vi "Sample 3 - Async Programming.vi"() -> ()   [LabVIEW 2016]
panel:
  in  "System Locator":string="usb:ix:0"
  in  "exit":bool
  out "Error":errorcluster
  out "Status B":T1(ring)
  out "Status A":T1(ring)
  in  "Channel B":u32
  in  "Channel A":u32
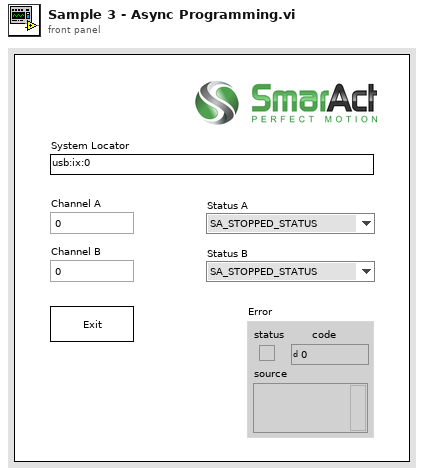
[diagram p1: front panel]
types:
  T1 = enum16{"SA_STOPPED_STATUS", "SA_STEPPING_STATUS", "SA_SCANNING_STATUS", "SA_HOLDING_STATUS", "SA_TARGET_STATUS", "SA_MOVE_DELAY_STATUS", "SA_CALIBRATING_STATUS", "SA_FINDING_REF_STATUS", "SA_OPENING_STATUS"}
  T2 = enum32{"SA_UNBUFFERED_OUTPUT", "SA_BUFFERED_OUTPUT"}
  T3 = typedef "mcsPacket.ctl" = cluster{"packetType":enum32{"SA_NO PACKET_TYPE", "SA_ERROR_ PACKET_TYPE", "SA_POSITION PACKET_TYPE", "SA_COMPLETED PACKET_TYPE", "SA_STATUS PACKET_TYPE", "SA_ANGLE_PACKET_TYPE", "SA_VOLTAGE_LEVEL_PACKET_TYPE", "SA_SENSOR_TYPE_PACKET_TYPE", "SA_SENSOR_ENABLED_PACKET_TYPE", "SA_END_EFFECTOR_TYPE_PACKET_TYPE", "SA_GRIPPER_OPENING_PACKET_TYPE", "SA_FORCE_PACKET_TYPE", "SA_MOVE_SPEED_PACKET_TYPE", "SA_PHYSICAL_POSITION_KNOWN_PACKET_TYPE", "SA_POSITION_LIMIT_PACKET_TYPE", "SA_ANGLE_LIMIT_PACKET_TYPE", "SA_SAFE_DIRECTION_PACKET_TYPE", "SA_SCALE_PACKET_TYPE", "SA_MOVE_ACCELERATION_PACKET_TYPE", "SA_CHANNEL_PROPERTY_PACKET_TYPE", "SA_CAPTURE_BUFFER_PACKET_TYPE", "SA_TRIGGERED_PACKET_TYPE"}, "channelIndex":u32, "data1":u32, "data2":i32, "data3":i32, "data4":u32}
  T4 = enum32{"SA_NO PACKET_TYPE", "SA_ERROR_ PACKET_TYPE", "SA_POSITION PACKET_TYPE", "SA_COMPLETED PACKET_TYPE", "SA_STATUS PACKET_TYPE", "SA_ANGLE_PACKET_TYPE", "SA_VOLTAGE_LEVEL_PACKET_TYPE", "SA_SENSOR_TYPE_PACKET_TYPE", "SA_SENSOR_ENABLED_PACKET_TYPE", "SA_END_EFFECTOR_TYPE_PACKET_TYPE", "SA_GRIPPER_OPENING_PACKET_TYPE", "SA_FORCE_PACKET_TYPE", "SA_MOVE_SPEED_PACKET_TYPE", "SA_PHYSICAL_POSITION_KNOWN_PACKET_TYPE", "SA_POSITION_LIMIT_PACKET_TYPE", "SA_ANGLE_LIMIT_PACKET_TYPE", "SA_SAFE_DIRECTION_PACKET_TYPE", "SA_SCALE_PACKET_TYPE", "SA_MOVE_ACCELERATION_PACKET_TYPE", "SA_CHANNEL_PROPERTY_PACKET_TYPE", "SA_CAPTURE_BUFFER_PACKET_TYPE", "SA_TRIGGERED_PACKET_TYPE"}
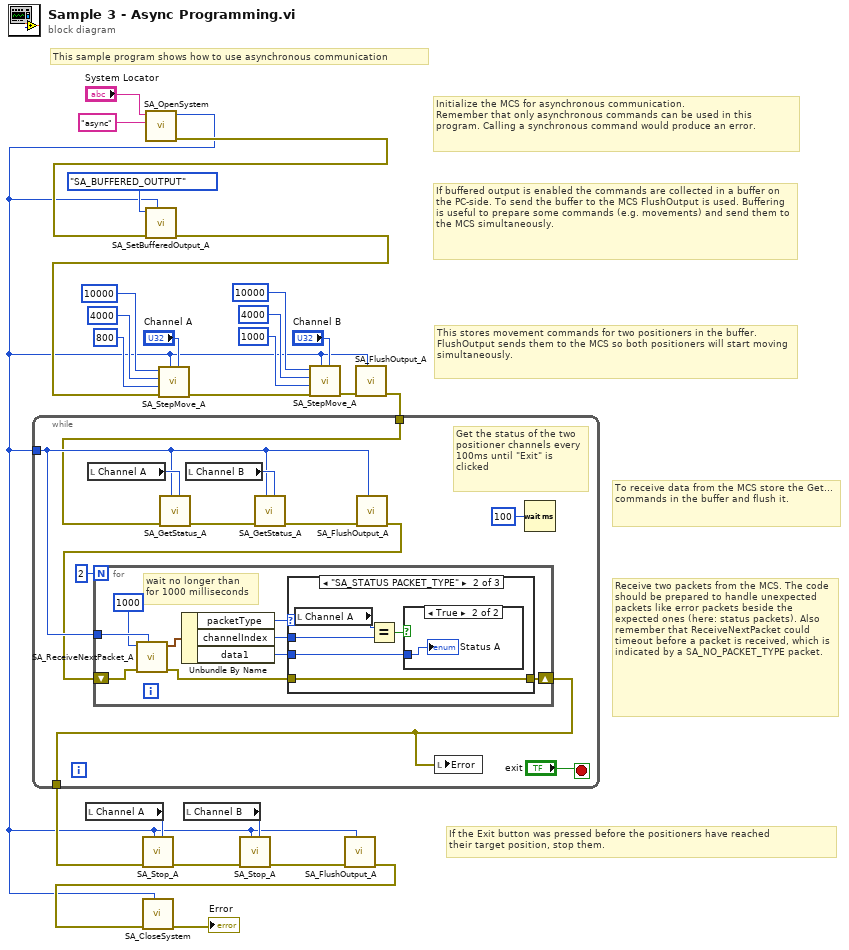
[diagram p0: block diagram]
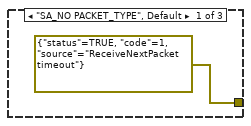
[diagram p2: hidden frame]
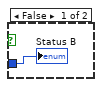
[diagram p3: hidden frame]
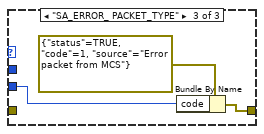
[diagram p4: hidden frame]
diagram:
  # "Initialize the MCS for asynchronous communication.\nRemember that only asynchronous commands can be used in this program. Calling a synchronous command would produce an error."
  # "If the Exit button was pressed before the positioners have reached\ntheir target position, stop them."
  # "Receive two packets from the MCS. The code should be prepared to handle unexpected packets like error packets beside the expected ones (here: status packets). Also remember that ReceiveNextPacket could timeout before a packet is received, which is indicated by a SA_NO_PACKET_TYPE packet."
  # "This sample program shows how to use asynchronous communication"
  # "To receive data from the MCS store the Get... commands in the buffer and flush it."
  # "This stores movement commands for two positioners in the buffer. FlushOutput sends them to the MCS so both positioners will start moving simultaneously."
  # "If buffered output is enabled the commands are collected in a buffer on the PC-side. To send the buffer to the MCS FlushOutput is used. Buffering is useful to prepare some commands (e.g. movements) and send them to the MCS simultaneously."
  n1 = local read "Channel A"() -> (w10:u32)
  n2 = call <vilib>:"SA_OpenSystem.vi"("options"="async", "systemLocator"="System Locator") -> ("error out"=w24:errorcluster, "systemIndexOut"=w1:u32)  [unwired: 8 in]
  n3 = call <vilib>:"SA_SetBufferedOutput_A.vi"("systemIndex"=w1, "error in (no error)"=w24, "mode"=T2."SA_BUFFERED_OUTPUT") -> ("error out"=w22:errorcluster)  [unwired: 8 in]
  n4 = call <vilib>:"SA_StepMove_A.vi"("channelIndex"="Channel A", "systemIndex"=w1, "error in (no error)"=w22, "frequency"=u32 800 ("steps"), "amplitude"=u32 4000 ("steps"), "steps"=10000) -> ("error out"=w20:errorcluster)  [unwired: 5 in]
  n5 = local read "Channel B"() -> (w9:u32)
  n6 = call <vilib>:"SA_StepMove_A.vi"("channelIndex"="Channel B", "systemIndex"=w1, "error in (no error)"=w20, "frequency"=u32 1000 ("steps"), "amplitude"=u32 4000 ("steps"), "steps"=10000) -> ("error out"=w18:errorcluster)  [unwired: 5 in]
  n7 = call <vilib>:"SA_FlushOutput_A.vi"("systemIndex"=w1, "error in (no error)"=w18) -> ("error out"=w4:errorcluster)  [unwired: 9 in]
  n8 = while {
    tunnel: w1 -> [w31]
    tunnel: [w26] -> w8
    tunnel: w4 -> [w27]
    stop <- "exit" stop-if-true
    # "Get the status of the two positioner channels every 100ms until \"Exit\" is clicked"
    n9 = local read "Channel A"() -> (w34:u32)
    n10 = call <vilib>:"SA_GetStatus_A.vi"("channelIndex"=w34, "systemIndex"=w31, "error in (no error)"=w27) -> ("error out"=w35:errorcluster)  [unwired: 8 in]
    n11 = local read "Channel B"() -> (w33:u32)
    n12 = call <vilib>:"SA_GetStatus_A.vi"("channelIndex"=w33, "systemIndex"=w31, "error in (no error)"=w35) -> ("error out"=w32:errorcluster)  [unwired: 8 in]
    n13 = call <vilib>:"SA_FlushOutput_A.vi"("systemIndex"=w31, "error in (no error)"=w32) -> ("error out"=w30:errorcluster)  [unwired: 9 in]
    n14 = for {
      N: 2 -> [_]
      tunnel: w31 -> [w44]
      shift-right: [w36] -> w26
      shift-left: w30 -> [w42]
      # "wait no longer than\nfor 1000 milliseconds"
      n15 = call <vilib>:"SA_ReceiveNextPacket_A.vi"("systemIndex"=w44, "error in (no error)"=w42, "timeout"=u32 1000) -> ("error out"=w37:errorcluster, "packet"=w40:T3)  [unwired: 7 in]
      n16 = Unbundle By Name(w40) -> ("packetType"=w41:T4, "channelIndex"=w39:u32, "data1"=w38:u32)
      n17 = case shown="\"SA_STATUS PACKET_TYPE\"" w41 {
        tunnel: w39 -> [_ w50 _]
        tunnel: w38 -> [_ w47 w53]
        tunnel: w37 -> [_ w46 _]
        tunnel: [errorcluster {"status"=TRUE, "code"=1, "source"="ReceiveNextPacket timeout"} ("error out") w46 w54] -> w36
        frame "SA_NO PACKET_TYPE", Default {
        }
        frame "SA_STATUS PACKET_TYPE" {
          n18 = local read "Channel A"() -> (w49:u32)
          n19 = Equal?(x=w49, y=w50) -> (x = y?=w48:bool)
          n20 = case shown="True" w48 {
            tunnel: w47 -> [w51 w52]
            frame False {
              "Status B" <- w51
            }
            frame True {
              "Status A" <- w52
            }
          }
        }
        frame "SA_ERROR_ PACKET_TYPE" {
          n21 = Bundle By Name(cluster=errorcluster {"status"=TRUE, "code"=1, "source"="Error packet from MCS"} ("error out"), "code"=w53) -> (w54:errorcluster)
        }
      }
    }
    n22 = local write "Error"(w26) -> ()
    n23 = Wait (ms)(milliseconds to wait=u32 100) -> ()  [unwired: 1 out]
  }
  n24 = call <vilib>:"SA_Stop_A.vi"("channelIndex"=w10, "systemIndex"=w1, "error in (no error)"=w8) -> ("error out"=w7:errorcluster)  [unwired: 8 in]
  n25 = call <vilib>:"SA_Stop_A.vi"("channelIndex"=w9, "systemIndex"=w1, "error in (no error)"=w7) -> ("error out"=w6:errorcluster)  [unwired: 8 in]
  n26 = call <vilib>:"SA_FlushOutput_A.vi"("systemIndex"=w1, "error in (no error)"=w6) -> ("error out"=w5:errorcluster)  [unwired: 9 in]
  n27 = call <vilib>:"SA_CloseSystem.vi"("systemIndex"=w1, "error in (no error)"=w5) -> ("error out"=→"Error":errorcluster)  [unwired: 9 in]
